vi "Get_data.vi"() -> (0 "EOF? and Error status":bool, 6 "Block Header":string)   [LabVIEW 2015]
uses:
  Controls/Block_start_and_end.ctl
  Globals/Meas_global.vi
  Globals/Trav_pos_global.vi
  Globals/LDA_meas_global_1.vi
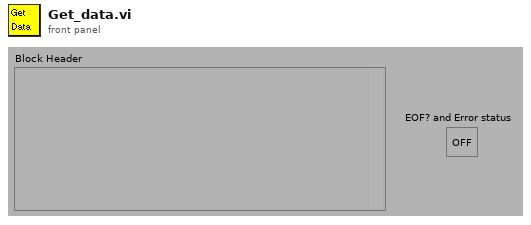
[diagram p1: front panel]
types:
  T1 = typedef "Block_start_and_end.ctl" = cluster{"Started":dbl, "Ended":dbl, "Analogue Frequency Hz":dbl}
  T2 = typedef "Post_Process.ctl" = enum16{"Take New Data", "Post Process Raw Data File"}
  T3 = typedef "PWA_Data.ctl" = enum16{"No PWA Data", "One Ch PWA"}
  T4 = typedef "BSA_Type.ctl" = enum16{"57N11", "BSA F60"}
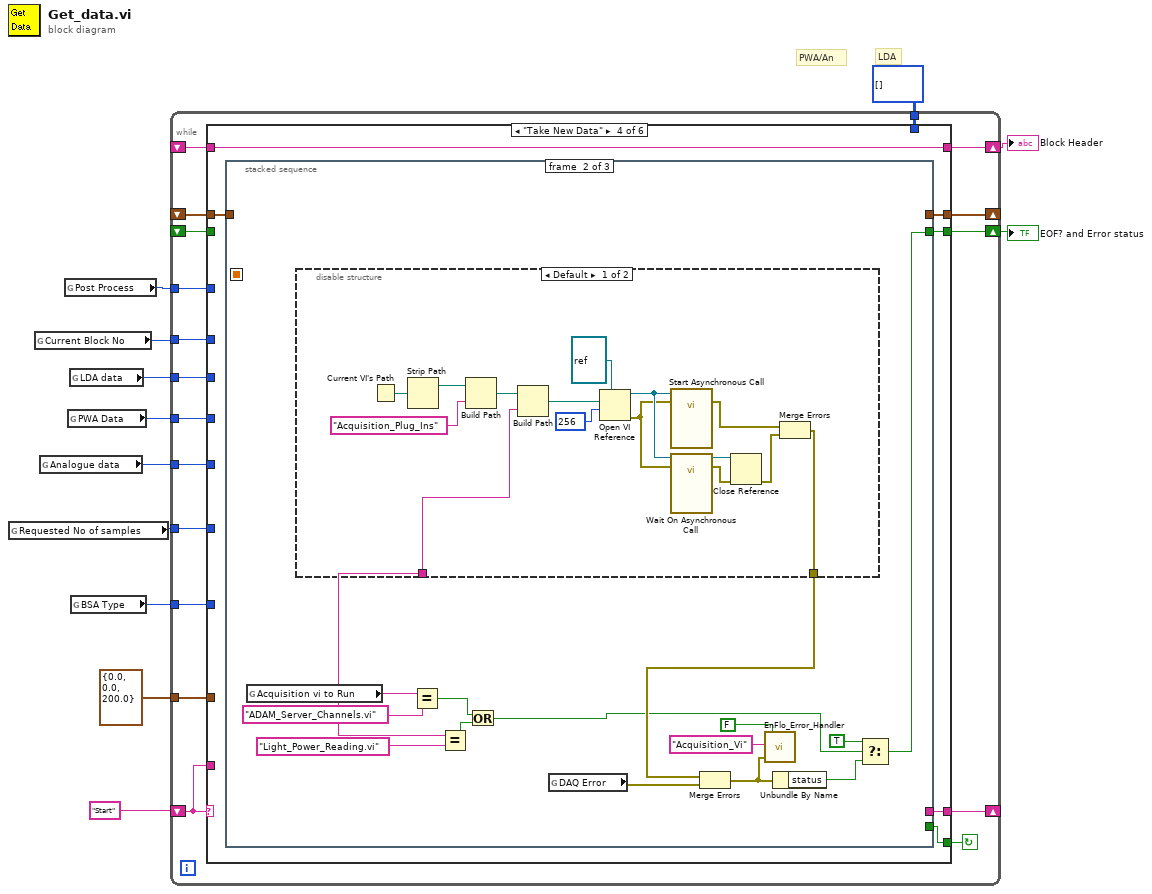
[diagram p0: block diagram]
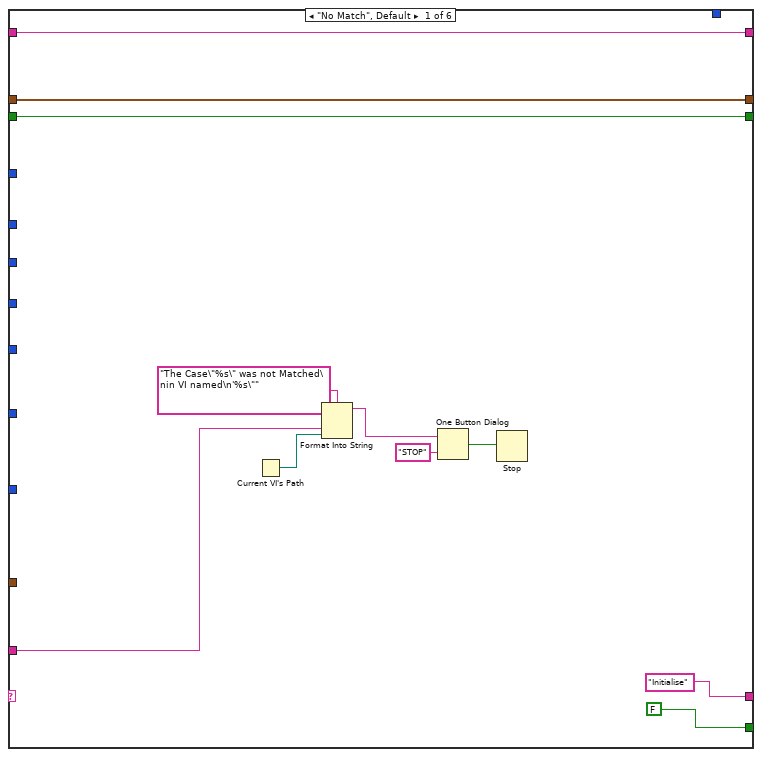
[diagram p2: hidden frame]
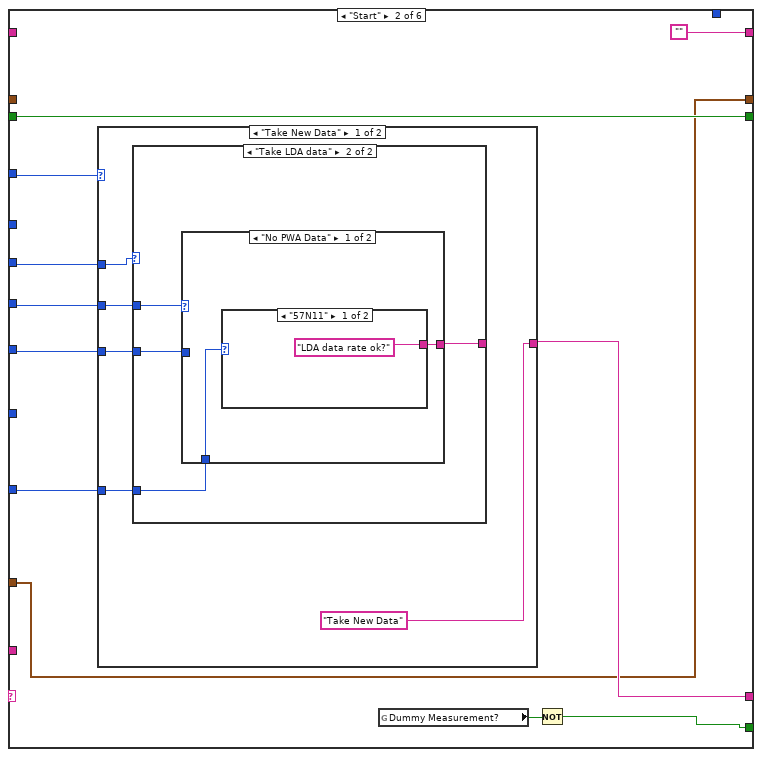
[diagram p3: hidden frame]
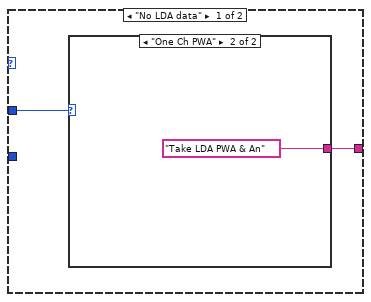
[diagram p4: hidden frame]
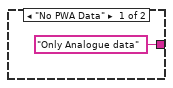
[diagram p5: hidden frame]
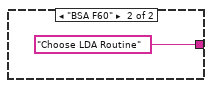
[diagram p6: hidden frame]
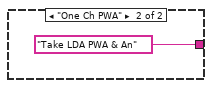
[diagram p7: hidden frame]
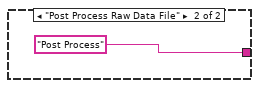
[diagram p8: hidden frame]
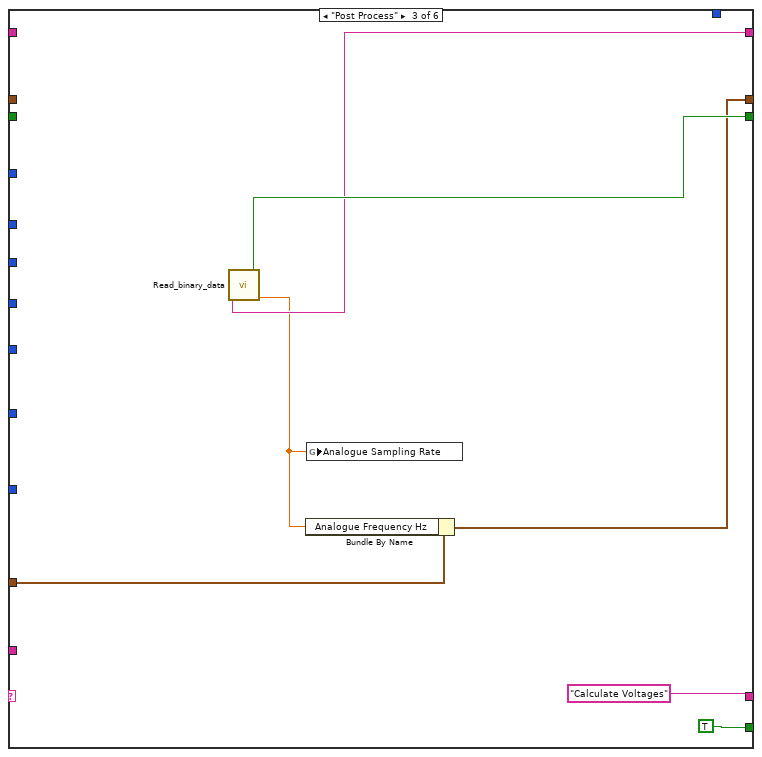
[diagram p9: hidden frame]
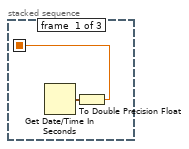
[diagram p10: hidden frame]
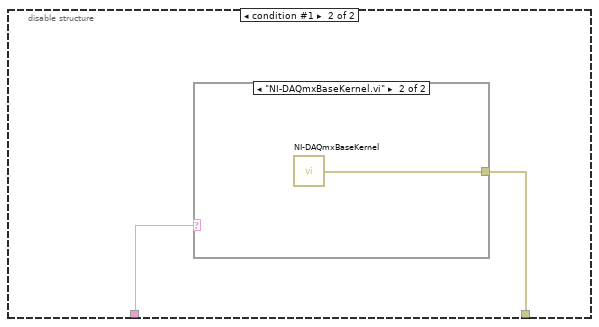
[diagram p11: hidden frame]
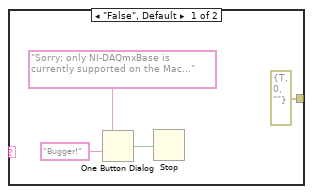
[diagram p12: hidden frame]
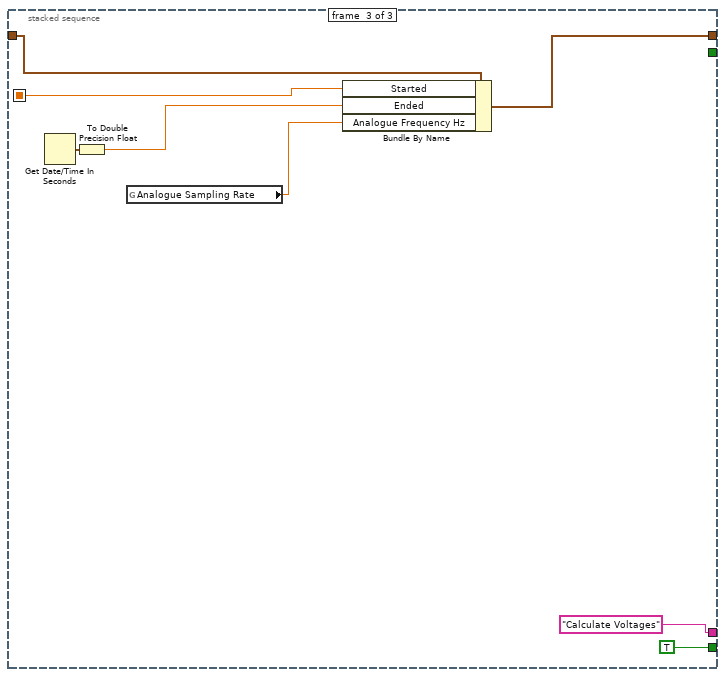
[diagram p13: hidden frame]
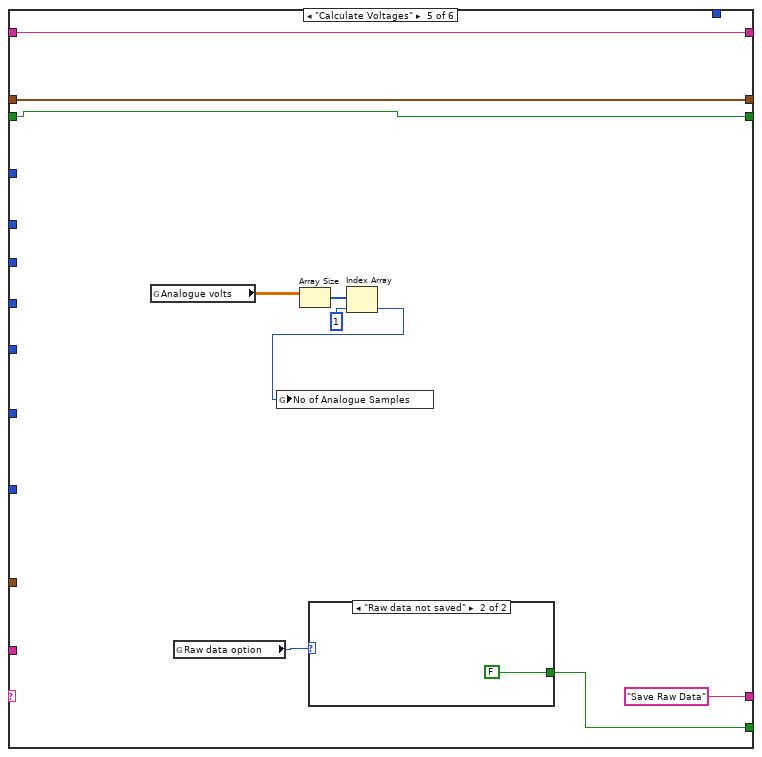
[diagram p14: hidden frame]
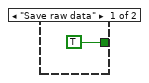
[diagram p15: hidden frame]
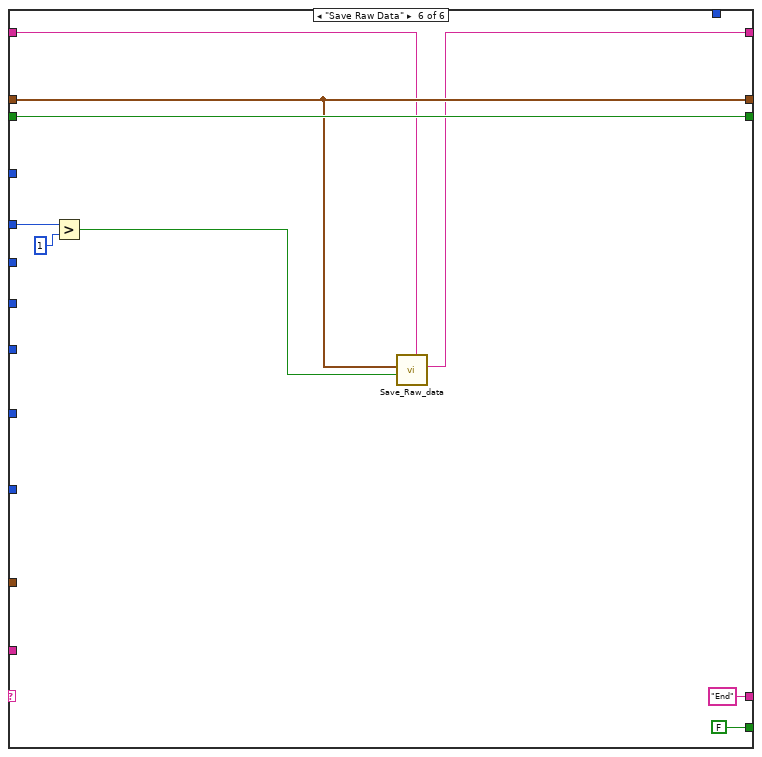
[diagram p16: hidden frame]
diagram:
  # "LDA"
  # "PWA/An"
  n1 = global read "Meas_global.vi" "Requested No of samples"() -> (w8:i32)
  n2 = global read "Meas_global.vi" "Current Block No"() -> (w7:i32)
  n3 = global read "Meas_global.vi" "Analogue data"() -> (w6:enum16{"No Analogue data", "Take Analogue data"})
  n4 = global read "Meas_global.vi" "Post Process"() -> (w9:T2)
  n5 = global read "Meas_global.vi" "PWA Data"() -> (w4:T3)
  n6 = global read "Meas_global.vi" "LDA data"() -> (w5:enum16{"No LDA data", "Take LDA data"})
  n7 = global read "LDA_meas_global_1.vi" "BSA Type"() -> (w1:T4)
  n8 = while {
    shift-left: "Start" -> [w28]
    shift-right: [w29] -> _
    shift-right: [w27] -> _
    shift-left: _ -> [w26]
    shift-right: [w25] -> w11
    shift-left: _ -> [w24]
    tunnel: T1 {"Started"=0.0, "Ended"=0.0, "Analogue Frequency Hz"=200.0} ("Block Timings") -> [w23]
    tunnel: w9 -> [w22]
    tunnel: w8 -> [w21]
    tunnel: w7 -> [w20]
    tunnel: w6 -> [w19]
    tunnel: w5 -> [w18]
    tunnel: w4 -> [w17]
    tunnel: u16[][] [] ("LDA Binary output") -> [w16]
    tunnel: w1 -> [w15]
    shift-right: [w13] -> w2
    shift-left: _ -> [w14]
    stop <- w30 continue-if-true
    n9 = case shown="\"Take New Data\"" w28 {
      tunnel: [FALSE w42 TRUE w80 w136 FALSE] -> w30
      tunnel: ["Initialise" w50 "Calculate Voltages" w81 "Save Raw Data" "End"] -> w29
      tunnel: w28 -> [w36 _ _ _ _ _]
      tunnel: [w33 w44 w74 w82 w140 w150] -> w27
      tunnel: w26 -> [w33 _ _ w83 w140 w150]
      tunnel: [w31 w52 w75 w79 w139 w151] -> w25
      tunnel: w24 -> [w31 w52 _ _ w139 w151]
      tunnel: w23 -> [_ w44 w76 _ _ _]
      tunnel: w22 -> [_ w51 _ _ _ _]
      tunnel: w21 -> [_ _ _ _ _ _]
      tunnel: w20 -> [_ _ _ _ _ w145]
      tunnel: w19 -> [_ w49 _ _ _ _]
      tunnel: w18 -> [_ w48 _ _ _ _]
      tunnel: w17 -> [_ w47 _ _ _ _]
      tunnel: w16 -> [_ _ _ _ _ _]
      tunnel: w15 -> [_ w46 _ _ _ _]
      tunnel: [w32 "" w73 w84 w135 w147] -> w13
      tunnel: w14 -> [w32 _ _ w84 w135 w146]
      frame "No Match", Default {
        n10 = Current VI's Path() -> (path=w35:path)
        n11 = Format Into String(format string="The Case\"%s\" was not Matched\nin VI named\n'%s\"" ("Format String"), w36, w35) -> (resulting string=w39:string)  [unwired: 2 in, 1 out]
        n12 = One Button Dialog(message=w39, button name ("OK")="STOP") -> (true=w37:bool)
        n13 = Stop(stop? (T)=w37) -> ()
      }
      frame "Start" {
        n14 = case shown="\"Take New Data\"" w51 {
          tunnel: ["Take New Data" "Post Process"] -> w50
          tunnel: w49 -> [w57 _]
          tunnel: w48 -> [w56 _]
          tunnel: w47 -> [w55 _]
          tunnel: w46 -> [w54 _]
          frame "Take New Data" {
            n15 = case shown="\"Take LDA data\"" w56 {
              tunnel: w57 -> [_ w63]
              tunnel: [w58 w65] -> _
              tunnel: w55 -> [w59 w64]
              tunnel: w54 -> [_ w62]
              frame "No LDA data" {
                n16 = case shown="\"One Ch PWA\"" w59 {
                  tunnel: ["Only Analogue data" "Take LDA PWA & An"] -> w58
                  frame "No PWA Data" {
                  }
                  frame "One Ch PWA" {
                  }
                }
              }
              frame "Take LDA data" {
                n17 = case shown="\"No PWA Data\"" w64 {
                  tunnel: [w66 "Take LDA PWA & An"] -> w65
                  tunnel: w63 -> [_ _]
                  tunnel: w62 -> [w67 _]
                  frame "No PWA Data" {
                    n18 = case shown="\"57N11\"" w67 {
                      tunnel: ["LDA data rate ok?" "Choose LDA Routine"] -> w66
                      frame "57N11" {
                      }
                      frame "BSA F60" {
                      }
                    }
                  }
                  frame "One Ch PWA" {
                  }
                }
              }
            }
          }
          frame "Post Process Raw Data File" {
          }
        }
        n19 = global read "Trav_pos_global.vi" "Dummy Measurement?"() -> (w43:bool)
        n20 = Not(x=w43) -> (.not. x?=w42:bool)
      }
      frame "Post Process" {
        n21 = call "Read_binary_data.vi"() -> ("Analogue Frequency Hz"=w72:dbl, "EOF?"=w75:bool, "Block Header"=w73:string)  [unwired: 7 out]
        n22 = Bundle By Name(cluster=w76, "Analogue Frequency Hz"=w72) -> (w74:T1)
        n23 = global write "Meas_global.vi" "Analogue Sampling Rate"(w72) -> ()
      }
      frame "Take New Data" {
        n24 = stacked-sequence {
          seq-local: [w85 _ _] -> [_ _ w128]
          tunnel: w83 -> [_ _ w129]
          tunnel: [_ _ w126] -> w82
          tunnel: [_ _ "Calculate Voltages"] -> w81
          tunnel: [_ _ TRUE] -> w80
          tunnel: [_ w94 _] -> w79
          frame #0 {
            n25 = Get Date/Time In Seconds() -> (seconds since 1Jan1904=w86:timestamp)
            n26 = To Double Precision Float(number=w86) -> (double precision float=w85:dbl)
          }
          frame #1 {
            n27 = global read "Meas_global.vi" "Acquisition vi to Run"() -> (w91:string)
            n28 = disable-structure shown="Default" {
              disable-tunnel: w91 -> [w115 w117]
              disable-tunnel: [w101 w116] -> w92
              frame condition #0 (active) {
                n29 = Current VI's Path() -> (path=w114:path)
                n30 = Strip Path(path=w114) -> (stripped path=w112:path)  [unwired: 1 out]
                n31 = Build Path(base path=w112, name or relative path="Acquisition_Plug_Ins") -> (appended path=w111:path)
                n32 = Build Path(base path=w111, name or relative path=w115) -> (appended path=w110:path)
                n33 = Open VI Reference(type specifier VI Refnum (for type only)=refnum<vi> refnum, vi path=w110, options=256) -> (vi reference=w108:refnum<vi>, error out=w107:errorcluster)  [unwired: 3 in]
                n34 = call-by-ref "Start Asynchronous Call"(reference=w108, error in=w107) -> (error out=w103:errorcluster)  [unwired: 1 in, 2 out]
                n35 = call-by-ref "Wait On Asynchronous Call"(reference=w108, error in=w107) -> (reference out=w105:refnum<vi>, error out=w104:errorcluster)  [unwired: 1 in, 1 out]
                n36 = Close Reference(reference=w105, error in (no error)=w104) -> (error out=w102:errorcluster)
                n37 = Merge Errors(w103, w102) -> (w101:errorcluster)
              }
              frame condition #1 {
                n38 = case shown="\"NI-DAQmxBaseKernel.vi\"" w117 {
                  tunnel: [errorcluster {"status"=TRUE, "code"=0, "source"=""} ("Error Out") w122] -> w116
                  frame "False", Default {
                    n39 = One Button Dialog(message="Sorry; only NI-DAQmxBase is currently supported on the Mac...", button name ("OK")="Bugger!") -> (true=w119:bool)
                    n40 = Stop(stop? (T)=w119) -> ()
                  }
                  frame "NI-DAQmxBaseKernel.vi" {
                    n41 = call "NI-DAQmxBaseKernel.vi"() -> ("Error Out"=w122:errorcluster)  [unwired: 1 in]
                  }
                }
              }
            }
            n42 = Equal?(x=w91, y="ADAM_Server_Channels.vi" ("Acquisition vi to Run")) -> (x = y?=w88:bool)
            n43 = Equal?(x=w91, y="Light_Power_Reading.vi" ("Acquisition vi to Run")) -> (x = y?=w89:bool)
            n44 = Or(x=w88, y=w89) -> (x .or. y?=w87:bool)
            n45 = global read "Meas_global.vi" "DAQ Error"() -> (w97:errorcluster)
            n46 = Merge Errors(w92, w97) -> (w96:errorcluster)
            n47 = call "EnFlo_Error_Handler.vi"("error in (no error)"=w96, "Error Type"="Acquisition_Vi", "Dialog Box (T)"=FALSE) -> ()  [unwired: 3 out]
            n48 = Unbundle By Name(w96) -> ("status"=w95:bool)
            n49 = Select(t=TRUE, s=w87, f=w95) -> (s? t:f=w94:bool)
          }
          frame #2 {
            n50 = Get Date/Time In Seconds() -> (seconds since 1Jan1904=w130:timestamp)
            n51 = To Double Precision Float(number=w130) -> (double precision float=w127:dbl)
            n52 = global read "Meas_global.vi" "Analogue Sampling Rate"() -> (w123:dbl)
            n53 = Bundle By Name(cluster=w129, "Started"=w128, "Ended"=w127, "Analogue Frequency Hz"=w123) -> (w126:T1)
          }
        }
      }
      frame "Calculate Voltages" {
        n54 = global read "Meas_global.vi" "Analogue volts"() -> (w131:dbl[][])
        n55 = global read "Meas_global.vi" "Raw data option"() -> (w138:enum16{"Save raw data", "Raw data not saved"})
        n56 = Array Size(array=w131) -> (size(s)=w132:i32[])
        n57 = case shown="\"Raw data not saved\"" w138 {
          tunnel: [TRUE FALSE] -> w136
          frame "Save raw data" {
          }
          frame "Raw data not saved" {
          }
        }
        n58 = Index Array(array=w132, index=1) -> (element=w134:i32)
        n59 = global write "Meas_global.vi" "No of Analogue Samples"(w134) -> ()
      }
      frame "Save Raw Data" {
        n60 = Greater?(x=w145, y=1) -> (0:w143:bool)
        n61 = call "Save_Raw_data.vi"("Add to Block Header"=w146, "append to file? (new file:F)"=w143, "Block Timings"=w150) -> ("Block Header"=w147:string)  [unwired: 6 in]
      }
    }
  }
  "EOF? and Error status" <- w11
  "Block Header" <- w2
